vi "plunge_mode.vi"() -> ()   [LabVIEW 2019]
uses:
  <userlib>/Nanonis Prog Interface V5/Nanonis Prog Interface.lvlib
  <userlib>/Haptic Prog Interface/Haptic Prog Interface.lvlib
panel:
  out "Zthresh (m)":dbl
  in  "Fine Adj":dbl=1.0
  in  "Rough Adj.":dbl
  out "force":dbl
  out "Z Write (m) 2":dbl
  in  "Z Write?":bool
  in  "Save":bool
  in  "# Sample Points":i32=16384
  out "Signal value":sgl format="%#_6p"
  out "Z Write (m)":dbl
  in  "Upper Limit (mm)":dbl=50.0
  in  "Lower Limit (mm)":dbl=-40.0
  in  "Upper Limit (nm)":dbl=1.0
  in  "Lower Limit (nm)":dbl
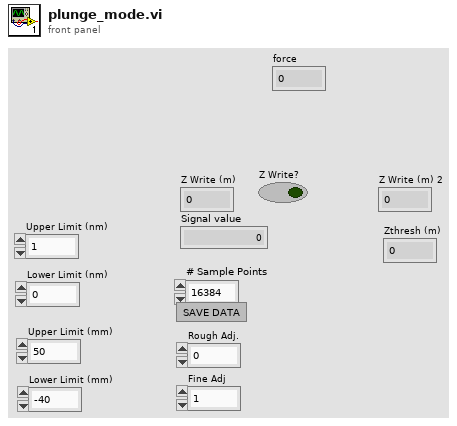
[diagram p1: front panel]
types:
  T1 = cluster{"Fx (N)":dbl, "Fy (N)":dbl, "Fz (N)":dbl}
  T2 = cluster{"x (mm)":dbl, "y (mm)":dbl, "z (mm)":dbl}
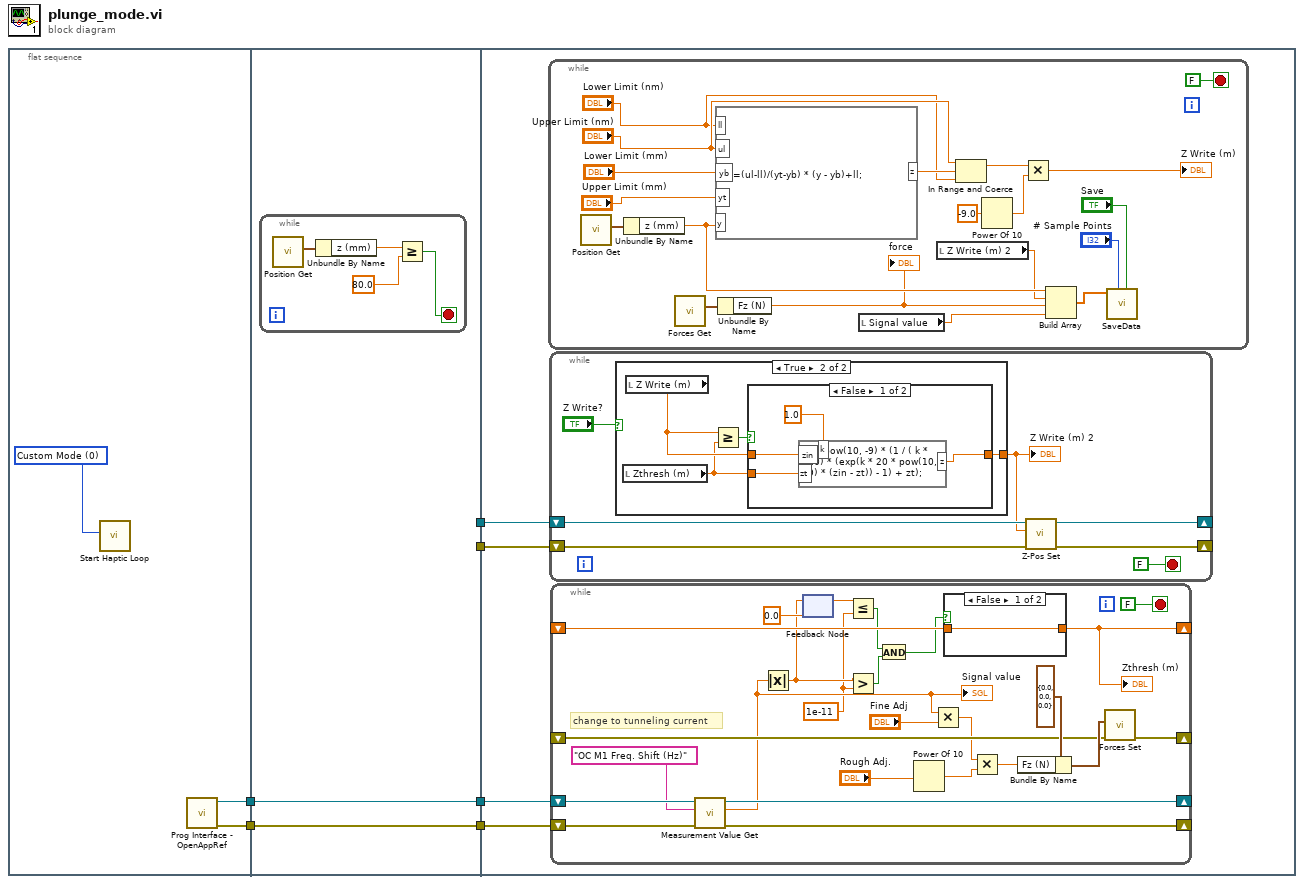
[diagram p0: block diagram]
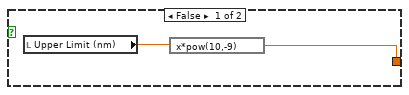
[diagram p2: hidden frame]
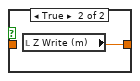
[diagram p4: hidden frame]
diagram:
  n1 = flat-sequence {
    tunnel: [w9] -> w6
    tunnel: [w8] -> w3
    tunnel: [w11] -> w5
    tunnel: [w10] -> w4
    tunnel: [w11] -> w2
    tunnel: [w10] -> w1
    tunnel: w3 -> [w10]
    tunnel: w6 -> [w11]
    tunnel: w5 -> [w19]
    tunnel: w4 -> [w18]
    tunnel: w2 -> [w17]
    tunnel: w1 -> [w16]
    frame #0 {
      w7 = u16 0 items=["Custom Mode", "Read Mode", "Write Mode"] ("Mode Selection")
      n2 = call <userlib>:"Start Haptic Loop.vi"("Mode Selection"=w7) -> ()  [unwired: 10 in, 1 out]
      n3 = call <userlib>:"Prog Interface - OpenAppRef.vi"() -> ("Error out"=w8:errorcluster, "Application reference"=w9:refnum<vi>)  [unwired: 6 in]
    }
    frame #1 {
      n4 = while {
        stop <- w14 stop-if-true
        n5 = call <userlib>:"Position Get.vi"() -> ("Position"=w13:T2)  [unwired: 10 in, 1 out]
        n6 = Unbundle By Name(w13) -> ("z (mm)"=w12:dbl)
        n7 = Greater Or Equal?(x=w12, y=80.0) -> (x >= y?=w14:bool)
      }
    }
    frame #2 {
      n8 = while {
        stop <- FALSE stop-if-true
        n9 = call <userlib>:"Position Get.vi"() -> ("Position"=w69:T2)  [unwired: 10 in, 1 out]
        n10 = Unbundle By Name(w69) -> ("z (mm)"=w68:dbl)
        n11 = call <userlib>:"Forces Get.vi"() -> ("Force (N)"=w67:T1)  [unwired: 10 in, 1 out]
        n12 = formula code="z =(ul-ll)/(yt-yb) * (y - yb)+ll;"("ll"="Lower Limit (nm)", "ul"="Upper Limit (nm)", "yb"="Lower Limit (mm)", "yt"="Upper Limit (mm)", "y"=w68) -> ("z"=w79:dbl)
        n13 = Unbundle By Name(w67) -> ("Fz (N)"=w66:dbl)
        "force" <- w66
        n14 = local read "Signal value"() -> (w72:sgl)
        n15 = local read "Z Write (m) 2"() -> (w65:dbl)
        n16 = In Range and Coerce(upper limit="Upper Limit (nm)", x=w79, lower limit="Lower Limit (nm)") -> (coerced(x)=w75:dbl)  [unwired: 1 out]
        n17 = Power Of 10(x=-9.0) -> (10^x=w80:dbl)
        n18 = Multiply(x=w75, y=w80) -> (x*y=→"Z Write (m)":dbl)
        n19 = Build Array(w68, w65, w66, w72) -> (w71:dbl[])
        n20 = call "SaveData.vi"("Save"="Save", "# Sample Points"="# Sample Points", "Data"=w71) -> ()  [unwired: 9 in]
      }
      n21 = while {
        shift-right: [w22] -> _
        shift-left: w17 -> [w24]
        shift-right: [w21] -> _
        shift-left: w16 -> [w23]
        stop <- FALSE stop-if-true
        n22 = case shown="True" "Z Write?" {
          tunnel: [w27 w31] -> w20
          frame False {
            n23 = local read "Upper Limit (nm)"() -> (w28:dbl)
            n24 = expression code="x*pow(10,-9)"(w28) -> (w27:dbl)
          }
          frame True {
            n25 = local read "Zthresh (m)"() -> (w29:dbl)
            n26 = local read "Z Write (m)"() -> (w30:dbl)
            n27 = Greater Or Equal?(x=w30, y=w29) -> (x >= y?=w32:bool)
            n28 = case shown="False" w32 {
              tunnel: w30 -> [w36 w37]
              tunnel: [w34 w37] -> w31
              tunnel: w29 -> [w35 _]
              frame False {
                n29 = formula code="z =pow(10, -9) * (1 / ( k * 20) * (exp(k * 20 * pow(10, 9) * (zin - zt)) - 1) + zt);"("zt"=w35, "zin"=w36, "k"=1.0 ("input variable")) -> ("z"=w34:dbl)
              }
              frame True {
              }
            }
          }
        }
        "Z Write (m) 2" <- w20
        n30 = call <userlib>:"Z-Pos Set.vi"("error in (no error)"=w23, "Z position (m)"=w20, "Application ref in"=w24) -> ("error out"=w21:errorcluster, "Application ref out"=w22:refnum<vi>)  [unwired: 7 in]
      }
      n31 = while {
        shift-right: [w59] -> _
        shift-left: w19 -> [w61]
        shift-right: [w58] -> _
        shift-left: w18 -> [w60]
        shift-right: [w54] -> _
        shift-left: _ -> [w53]
        shift-right: [w47] -> _
        shift-left: _ -> [w46]
        stop <- FALSE stop-if-true
        w39 = 1e-11 ("y")
        # "change to tunneling current"
        n32 = call <userlib>:"Measurement Value Get.vi"("error in (no error)"=w60, "Signal Name"="OC M1 Freq. Shift (Hz)", "Application ref in"=w61) -> ("error out"=w58:errorcluster, "Measurement value"=w44:sgl, "Application ref out"=w59:refnum<vi>)  [unwired: 5 in]
        "Signal value" <- w44
        n33 = Absolute Value(x=w44) -> (abs(x)=w40:sgl)
        n34 = feedback-in #1(w40) -> ()
        n35 = feedback #1(sgl 0.0 ("Measurement value")) -> (w41:sgl)
        n36 = Less Or Equal?(x=w41, y=w39) -> (x <= y?=w42:bool)
        n37 = Greater?(x=w40, y=w39) -> (0:w38:bool)
        n38 = And(x=w42, y=w38) -> (x .and. y?=w45:bool)
        n39 = Power Of 10(x="Rough Adj.") -> (10^x=w50:dbl)
        n40 = Multiply(x=w44, y="Fine Adj") -> (x*y=w49:dbl)
        n41 = case shown="False" w45 {
          tunnel: [w63 w64] -> w47
          tunnel: w46 -> [w63 _]
          frame False {
          }
          frame True {
            n42 = local read "Z Write (m)"() -> (w64:dbl)
          }
        }
        "Zthresh (m)" <- w47
        n43 = Multiply(x=w49, y=w50) -> (x*y=w52:dbl)
        n44 = Bundle By Name(cluster=T1 {"Fx (N)"=0.0, "Fy (N)"=0.0, "Fz (N)"=0.0} ("Force (N)"), "Fz (N)"=w52) -> (w55:T1)
        n45 = call <userlib>:"Forces Set.vi"("error in (no error)"=w53, "Force (N)"=w55) -> ("error out"=w54:errorcluster)  [unwired: 9 in]
      }
    }
  }
